vi "Mensaje_W_1 (SubVI).vi"(11 "iteration":i32) -> (3 "MSG W1":string)   [LabVIEW 2021, in "Control Vis.lvlib"]
uses:
  Control Vis.lvlib
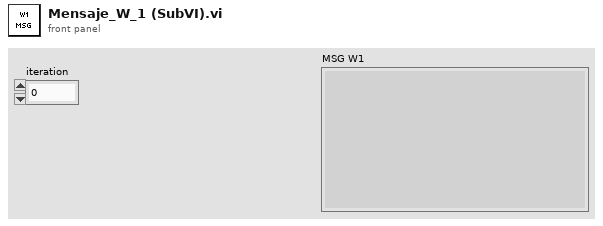
[diagram p1: front panel]
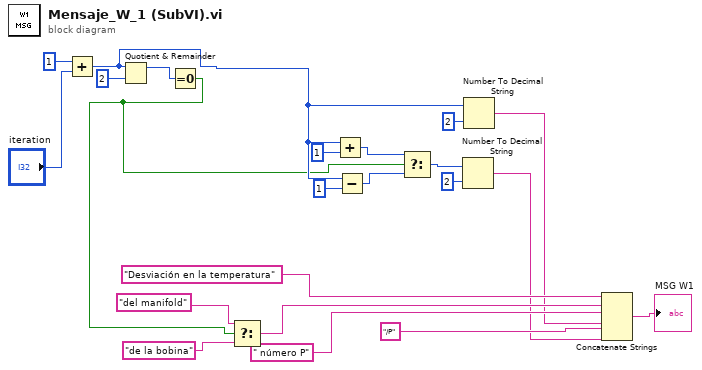
[diagram p0: block diagram]
diagram:
  n1 = Add(x=1, y="iteration") -> (x+y=w12:i32)
  n2 = Quotient & Remainder(x=w12, y=2) -> (x-y*floor(x/y)=w19:i32)  [unwired: 1 out]
  n3 = Equal To 0?(x=w19) -> (x = 0?=w10:bool)
  n4 = Select(t="del manifold" ("Descripcion"), s=w10, f="de la bobina" ("Descripcion")) -> (s? t:f=w20:string)
  n5 = Add(x=w12, y=1) -> (x+y=w9:i32)
  n6 = Subtract(x=w12, y=1) -> (x-y=w8:i32)
  n7 = Select(t=w9, s=w10, f=w8) -> (s? t:f=w7:i32)
  n8 = Number To Decimal String(number=w7, width (-)=i16 2) -> (decimal integer string=w4:string)
  n9 = Number To Decimal String(number=w12, width (-)=i16 2) -> (decimal integer string=w6:string)
  n10 = Concatenate Strings("Desviación en la temperatura" ("Descripcion"), w20, " número P" ("string"), w6, "/P" ("string"), w4) -> (→"MSG W1":string)
